vi "Binaryto TDMS converter11-30-2017.vi"(5 "Label header with scale information (on/ OFF)":bool, 7 "View TDMS Header information (on/ off)":bool, 9 "channel name":string="iq", 10 "original binary file Location":path, 11 "Scale Data":dbl) -> (1 "Converted Binary to TDMS location":path, 2 "Conversion Progress 2":dbl(slide) scale=0.0..100.0, 3 "Conversion Progress":dbl(slide)=inf scale=0.0..100.0)   [LabVIEW 2017]
uses:
  MainVI/GlobalVariableS.vi
  <vilib>/Utility/tdmsutil.llb/TDMS Create Scaling Information (Linear).vi
panel:
  in  "linear scale":T1={"Scale Data"=1.0000000000065512e-05, "y intercept"=0.0, "input source"=-1}
  in  "group name":string="vst"
  out "number of chuncks of elements read per second iteration":i32=2
  in  "first loop":bool
  out "number of chuncks of elements read per first  iteration":i32
  out "Original size (in bytes)":i64
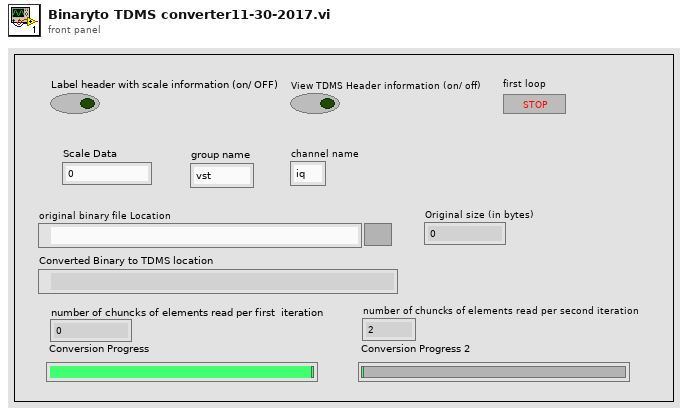
[diagram p1: front panel]
types:
  T1 = cluster{"Scale Data":dbl, "y intercept":dbl, "input source":i32}
  T2 = enum16{"open", "open or create", "create or replace", "create", "open (read-only)"}
  T3 = enum16{"big-endian, network order", "native, host order", "little-endian"}
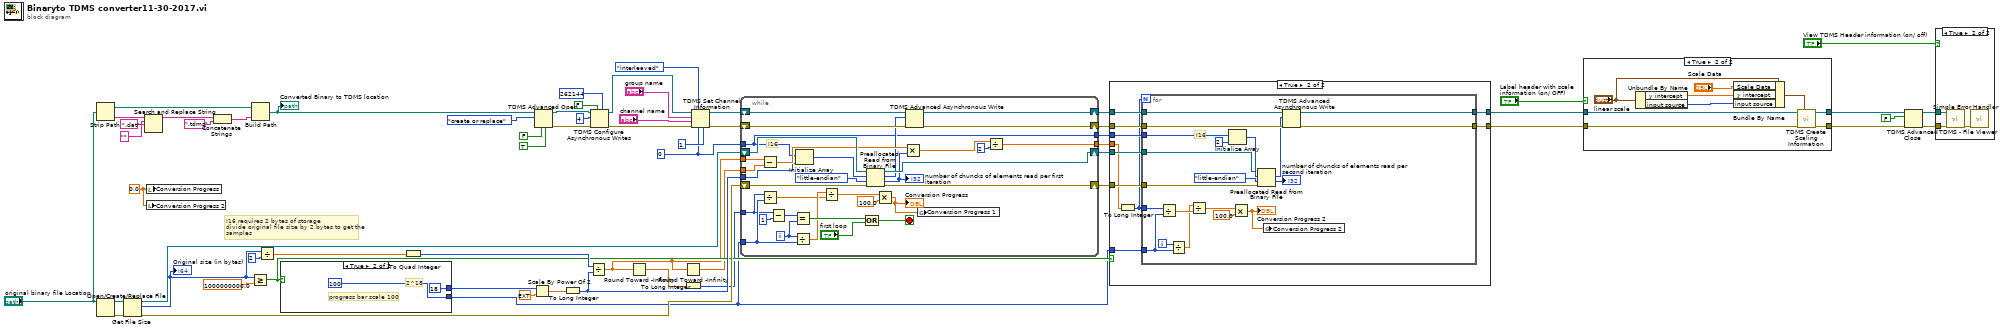
[diagram p0: block diagram]
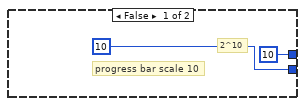
[diagram p4: hidden frame]
diagram:
  w1 = 0.0 ("Conversion Progress 2")
  w5 = i16 0 ("data type")
  # "I16 requires 2 bytes of storage\ndivide original file size by 2 bytes to get the \nsamples"
  n1 = Strip Path(path="original binary file Location") -> (stripped path=w14:path, name=w15:string)
  n2 = Open/Create/Replace File(file path (use dialog)="original binary file Location") -> (refnum out=w61:refnum<file>, error out=w60:errorcluster)  [unwired: 5 in, 1 out]
  n3 = Get File Size(file=w61, error in=w60) -> (refnum out=w49:refnum<file>, size (in bytes)=w36:i64, 0:w48:errorcluster)
  "Original size (in bytes)" <- w36
  n4 = Search and Replace String(input string=w15, search string=".dat", replace string="" ("replace string (\"\")")) -> (result string=w18:string)  [unwired: 5 in, 3 out]
  n5 = local write "Conversion Progress 2"(w1) -> ()
  n6 = local write "Conversion Progress"(w1) -> ()
  n7 = Concatenate Strings(w18, ".tdms" ("string")) -> (w19:string)
  n8 = Greater Or Equal?(x=w36, y=1000000000.0) -> (x >= y?=w33:bool)
  n9 = Build Path(base path=w14, name or relative path=w19) -> (appended path=w2:path)
  "Converted Binary to TDMS location" <- w2
  n10 = Divide(x=w36, y=2) -> (x/y=w55:dbl)
  n11 = case shown="True" w33 {
    tunnel: [10 ("2^x 2") 18 ("2^x")] -> w52
    tunnel: [10 ("y") 100 ("y")] -> w3
    frame False {
      # "progress bar scale 10"
      # "2^10"
    }
    frame True {
      # "progress bar scale 100"
      # "2^18"
    }
  }
  n12 = To Quad Integer(1:w55) -> (0:w46:i64)
  n13 = Scale By Power Of 2(n=w52, x=ext 1.0) -> (x*2^n=w53:ext)
  n14 = TDMS Advanced Open(4:TRUE ("disable buffering (F)"), 6:FALSE ("disable buffering? (T)"), 10:T2."create or replace" ("operation (0:open)"), 11:w2) -> (0:w28:errorcluster, 3:w29:refnum<k34>)  [unwired: 1 in, 1 out]
  n15 = To Long Integer(number=w53) -> (32bit integer=w50:i32)
  n16 = Divide(x=w46, y=w50) -> (x/y=w20:dbl)
  n17 = TDMS Configure Asynchronous Writes(5:u32 262144 ("max write size"), 7:FALSE ("pre-allocate? (F)"), 8:w28, 10:u32 4 ("max asynchronous writes (4)"), 11:w29) -> (0:w31:errorcluster, 3:w30:refnum<k34>)  [unwired: 2 in]
  n18 = Round Toward -Infinity(1:w20) -> (0:w22:dbl)
  n19 = Round Toward -Infinity(1:w20) -> (0:w21:dbl)
  n20 = To Long Integer(number=w22) -> (32bit integer=w4:i32)
  n21 = TDMS Set Channel Information(4:u32 1 ("data type"), 6:w5, 7:enum16{"non-interleaved", "interleaved"}."interleaved" ("data layout (0:non-interleaved)"), 8:w31, 9:"channel name", 10:"group name", 11:w30) -> (0:w57:errorcluster, 3:w58:refnum<k34>)
  n22 = while {
    tunnel: w50 -> [w67]
    shift-right: [w97] -> w43
    shift-left: w48 -> [w90]
    shift-right: [w75] -> w45
    shift-left: w58 -> [w73]
    shift-right: [w76] -> w44
    shift-left: w57 -> [w74]
    shift-right: [w96] -> w42
    shift-left: w49 -> [w92]
    tunnel: w4 -> [w72]
    tunnel: w20 -> [w87]
    tunnel: w21 -> [w88]
    tunnel: [w83] -> w40
    tunnel: w3 -> [w77]
    tunnel: [w68] -> w7
    tunnel: w5 -> [w68]
    i -> [w82]
    stop <- w93 stop-if-true
    # "I16"
    n23 = Subtract(x=w87, y=w88) -> (x-y=w86:dbl)
    n24 = Divide(x=w72, y=w77) -> (x/y=w80:dbl)
    n25 = Subtract(x=w72, y=1) -> (x-y=w71:i32)
    n26 = Equal?(x=w71, y=w82) -> (x = y?=w94:bool)
    n27 = Divide(x=w82, y=w77) -> (x/y=w81:dbl)
    n28 = Initialize Array(w68, w67) -> (w91:i16[])
    n29 = Divide(x=w81, y=w80) -> (x/y=w79:dbl)
    n30 = Compound Arithmetic op=OR(w94, "first loop") -> (w93:bool)
    n31 = Preallocated Read from Binary File(4:w90, 5:T3."little-endian" ("byte order (0:big-endian, network order)"), 6:w91, 7:w92) -> (0:w97:errorcluster, 1:w89:i32, 2:w69:i16[], 3:w96:refnum<file>)
    "number of chuncks of elements read per first  iteration" <- w89
    n32 = Multiply(x=w79, y=100.0) -> (x*y=w66:dbl)
    "Conversion Progress" <- w66
    n33 = Multiply(x=w86, y=w89) -> (x*y=w85:dbl)
    n34 = TDMS Advanced Asynchronous Write(8:w74, 10:w69, 11:w73) -> (0:w76:errorcluster, 3:w75:refnum<k34>)
    n35 = global write "GlobalVariableS.vi" "Conversion Progress 1"(w66) -> ()
    n36 = Divide(x=w85, y=i16 2) -> (x/y=w83:dbl)
  }
  n37 = case shown="True" w33 {
    tunnel: w45 -> [w100 w110]
    tunnel: w44 -> [w99 w109]
    tunnel: w43 -> [_ w108]
    tunnel: w42 -> [_ w107]
    tunnel: w40 -> [_ w106]
    tunnel: [w99 w105] -> w11
    tunnel: [w100 w104] -> w10
    tunnel: w7 -> [_ w103]
    tunnel: w3 -> [_ w101]
    frame False {
    }
    frame True {
      n38 = To Long Integer(number=w106) -> (32bit integer=w102:i32)
      n39 = for {
        N: w102 -> [_]
        tunnel: w110 -> [w130]
        tunnel: w109 -> [w129]
        tunnel: w107 -> [w126]
        tunnel: w108 -> [w125]
        tunnel: [w122] -> w105
        tunnel: [w123] -> w104
        tunnel: w103 -> [w121]
        tunnel: w102 -> [w117]
        tunnel: w101 -> [w116]
        i -> [w118]
        # "I16"
        n40 = Divide(x=w117, y=w116) -> (x/y=w115:dbl)
        n41 = Divide(x=w118, y=w116) -> (x/y=w114:dbl)
        n42 = Divide(x=w114, y=w115) -> (x/y=w112:dbl)
        n43 = Initialize Array(w121, 2 ("dimension size")) -> (w128:i16[])
        n44 = Multiply(x=w112, y=100.0) -> (x*y=w111:dbl)
        "Conversion Progress 2" <- w111
        n45 = Preallocated Read from Binary File(4:w125, 5:T3."little-endian" ("byte order (0:big-endian, network order)"), 6:w128, 7:w126) -> (1:→"number of chuncks of elements read per second iteration":i32, 2:w120:i16[])  [unwired: 2 out]
        n46 = global write "GlobalVariableS.vi" "Conversion Progress 2"(w111) -> ()
        n47 = TDMS Advanced Asynchronous Write(8:w129, 10:w120, 11:w130) -> (0:w122:errorcluster, 3:w123:refnum<k34>)
      }
    }
  }
  n48 = case shown="True" "Label header with scale information (on/ OFF)" {
    tunnel: [w131 w141] -> w9
    tunnel: [w132 w140] -> w6
    tunnel: w11 -> [w131 w139]
    tunnel: w10 -> [w132 w138]
    frame False {
    }
    frame True {
      n49 = Unbundle By Name("linear scale") -> ("y intercept"=w137:dbl, "input source"=w136:i32)
      n50 = Bundle By Name(cluster="linear scale", "Scale Data"="Scale Data", "y intercept"=w137, "input source"=w136) -> (w134:T1)
      n51 = call-poly <vilib>:"TDMS Create Scaling Information.vi"("linear scale"=w134, "error in (no error)"=w139, "tdms file"=w138) -> ("error out"=w141:errorcluster, "tdms file out"=w140:refnum<k34>)  [unwired: 4 in, 3 out]
    }
  }
  n52 = TDMS Advanced Close(8:w9, 10:FALSE ("truncate file? (F)"), 11:w6) -> (0:w39:errorcluster, 3:w38:path)  [unwired: 1 in]
  n53 = case shown="True" "View TDMS Header information (on/ off)" {
    tunnel: w39 -> [_ w144]
    tunnel: w38 -> [_ w143]
    frame False {
    }
    frame True {
      n54 = call <vilib>:"TDMS - File Viewer.vi"("error in (no error)"=w144, "file path"=w143) -> ("error out"=w142:errorcluster)  [unwired: 4 in, 1 out]
      n55 = call <vilib>:"Simple Error Handler.vi"("error in (no error)"=w142) -> ()  [unwired: 4 in, 5 out]
    }
  }
